vi "ServoHostClaw.vi"(8 "error in":errorcluster, 9 "Angle (deg) Claw":dbl(slide) scale=-90.0..90.0, 11 "FPGA VI Reference In":T1) -> (0 "error out":errorcluster, 3 "FPGA VI Reference Out":T1)   [LabVIEW 2012]
uses:
  FPGA_ref.ctl
  <vilib>/Utility/error.llb/Error Cluster From Error Code.vi
  <vilib>/rvi/errors/niLvFpgaAdjustHostInterfaceError.vi
  <vilib>/rvi/interface/nirviReadWriteControl/nirviReadWriteControl.xnode
  NiFpgaLv.dll
  <vilib>/rvi/interface/Simulation/niFpgaSimulationCallBeginRW.vi
panel:
  out "pulse width (us)  2":i32
  in  "lower limit (Claw)":dbl=-65.0
  in  "upper limit (Claw)":dbl=25.0
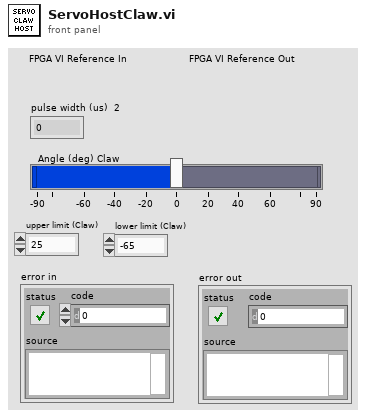
[diagram p1: front panel]
types:
  T1 = typedef "FPGA_ref.ctl" = refnum<k20>
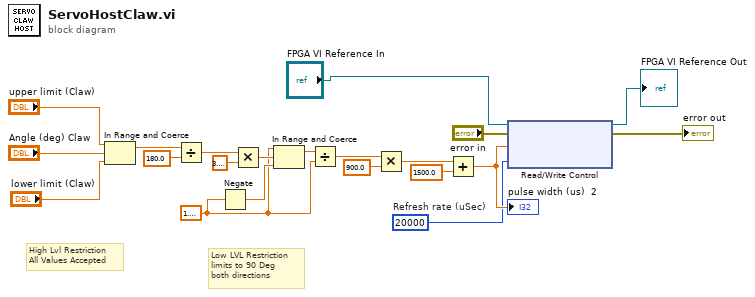
[diagram p0: block diagram]
diagram:
  w3 = 1.5707963267948966
  w5 = u32 20000  # Refresh rate (uSec)
  # "Low LVL Restriction\nlimits to 90 Deg \nboth directions"
  # "High Lvl Restriction\nAll Values Accepted"
  n1 = In Range and Coerce(upper limit="upper limit (Claw)", x="Angle (deg) Claw", lower limit="lower limit (Claw)") -> (coerced(x)=w19:dbl)  [unwired: 1 out]
  n2 = Divide(x=w19, y=180.0) -> (x/y=w15:dbl)
  n3 = Negate(x=w3) -> (-x=w14:dbl)
  n4 = Multiply(x=w15, y=3.141592653589793) -> (x*y=w16:dbl)
  n5 = In Range and Coerce(upper limit=w3, x=w16, lower limit=w14) -> (coerced(x)=w4:dbl)  [unwired: 1 out]
  n6 = Divide(x=w4, y=w3) -> (x/y=w13:dbl)
  n7 = Multiply(x=w13, y=900.0) -> (x*y=w10:dbl)
  n8 = Add(x=w10, y=1500.0) -> (x+y=w6:dbl)
  "pulse width (us)  2" <- w6
  n9 = xnode "Read/Write Control"("FPGA VI Reference In"="FPGA VI Reference In", "error in"="error in", "servo Claw"=w6, "Count(uSec) Claw"=w5) -> ("FPGA VI Reference Out"=→"FPGA VI Reference Out":T1, "error out"=→"error out":errorcluster)
